vi "Calculate conductance slim.vi"(0 "File or Folder Path":path=path "P:/expt/Leiden MNK/SA02836H.20170110/47", 5 "single ended?":bool=TRUE, 7 "index":T1={"N1"=18, "N2"=19, "N3"=4, "N4"=5, "V1"=8, "V2"=10, "V3"=10, "V4"=13, "CURRENT"=12, "Vsg"=1}, 9 "offset":i32, 11 "length":i32=1000) -> (4 "A vs D":cluster{dbl[], dbl[]}[](graph))   [LabVIEW 2016]
panel:
  in  "e^2/h":bool=TRUE
  out "Path":path=path "P:/expt/Leiden MNK/SA02836H.20170110/47/47 - Sweep axis 1,2 - 1/SA02836H.20170110.000034.itx"
  in  "file contains 2D data?":bool
  in  "recolor traces?":bool
  in  "B x name":string="Vsg (V)"
  in  "A y name":string="Conductance (S)"
  in  "Generate Folder Index File?":bool
  in  "pattern":string="*.itx"
  in  "Use Folder Index File?":bool
  # "CURRENT/(V1-V2)"
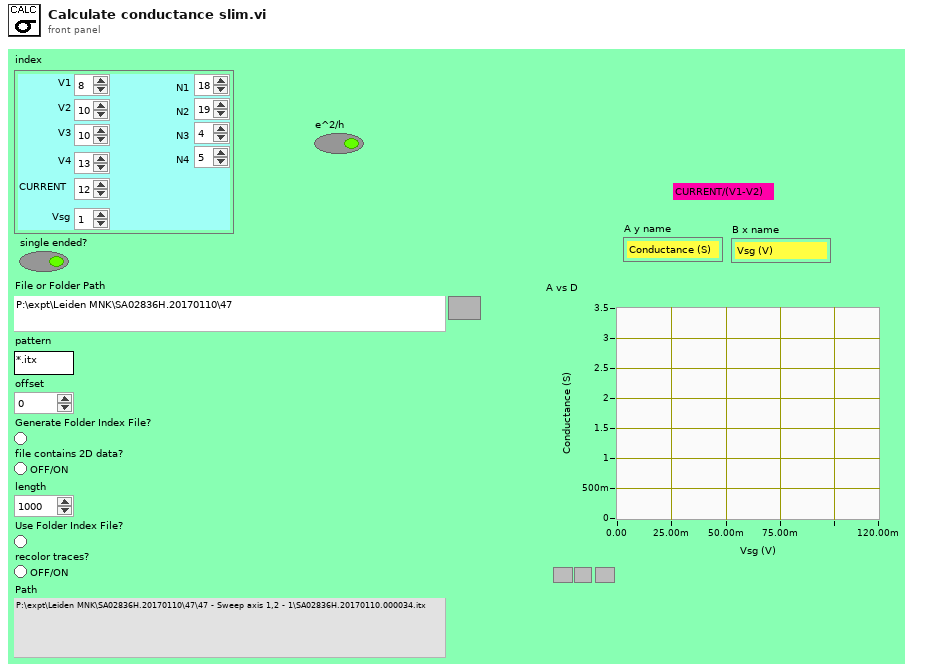
[diagram p1: front panel]
types:
  T1 = cluster{"N1":i32, "N2":i32, "N3":i32, "N4":i32, "V1":i32, "V2":i32, "V3":i32, "V4":i32, "CURRENT":i32, "Vsg":i32}
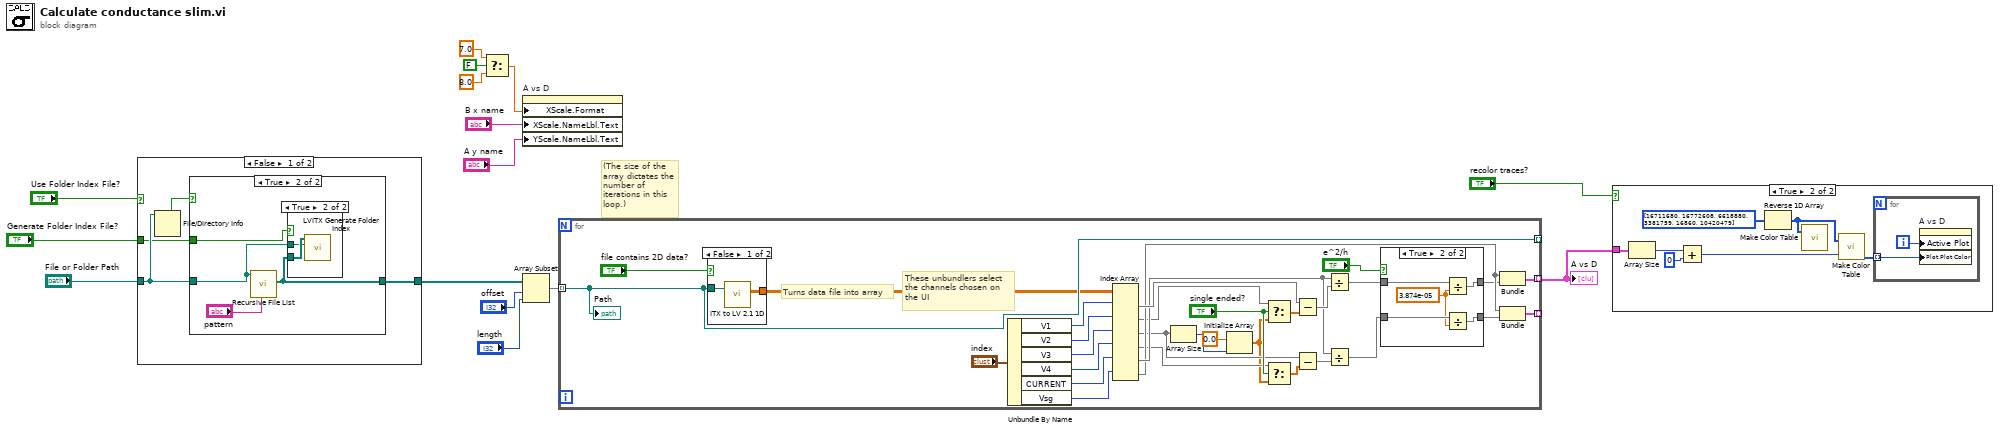
[diagram p0: block diagram]
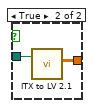
[diagram p4: hidden frame]
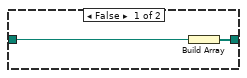
[diagram p5: hidden frame]
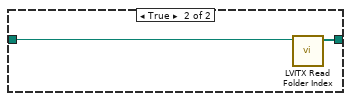
[diagram p7: hidden frame]
diagram:
  # "(The size of the array dictates the number of\niterations in this loop.)"
  n1 = case shown="False" "Use Folder Index File?" {
    tunnel: [w17 w28] -> w13
    tunnel: "File or Folder Path" -> [w19 w29]
    tunnel: "Generate Folder Index File?" -> [w16 _]
    frame False {
      n2 = File/Directory Info(path=w19) -> (directory=w18:bool)  [unwired: 1 in, 6 out]
      n3 = case shown="True" w18 {
        tunnel: [w21 w24] -> w17
        tunnel: w19 -> [w20 w23]
        tunnel: w16 -> [_ w22]
        frame False {
          n4 = Build Array(w20) -> (w21:path[])
        }
        frame True {
          n5 = call <vilib>:"Recursive File List.vi"("pattern"="pattern", "Folder Path"=w23) -> ("All Files in Dir"=w24:path[])  [unwired: 5 in, 4 out]
          n6 = case shown="True" w22 {
            tunnel: w24 -> [_ w27]
            tunnel: w23 -> [_ w26]
            frame False {
            }
            frame True {
              n7 = call <userlib>:"LVITX Generate Folder Index.vi"("File or Folder Path"=w26, "All Files in Dir"=w27) -> ()  [unwired: 10 in]
            }
          }
        }
      }
    }
    frame True {
      n8 = call <userlib>:"LVITX Read Folder Index.vi"("File or Folder Path"=w29) -> ("Array"=w28:path[])  [unwired: 10 in]
    }
  }
  n9 = Select(t=7.0, s=FALSE ("B is time?"), f=8.0) -> (s? t:f=w3:dbl)
  n10 = property on="A vs D" class="XYGraph (strict)"("XScale.Format"=w3, "XScale.NameLbl.Text"="B x name", "YScale.NameLbl.Text"="A y name") -> ()  [unwired: 2 in, 2 out]
  n11 = Array Subset(array=w13, index="offset", length="length") -> (w6:path[])
  n12 = for {
    tunnel: w6 -> [w60] mode=indexing
    tunnel: [w60] -> _ mode=indexing
    tunnel: [w31] -> w1 mode=indexing
    tunnel: [w47] -> _ mode=indexing
    # "These unbundlers select\nthe channels chosen on\nthe UI"
    # "Turns data file into array"
    n13 = case shown="False" "file contains 2D data?" {
      tunnel: [w68 w70] -> w52
      tunnel: w60 -> [w69 w71]
      frame False {
        n14 = call <userlib>:"ITX to LV 2.1 1D.vi"("file (use dialog)"=w69) -> ("1D arrays"=w68:dbl[][])  [unwired: 2 in, 2 out]
      }
      frame True {
        n15 = call <userlib>:"ITX to LV 2.1.vi"("file (use dialog)"=w71) -> ("1D arrays"=w70:dbl[][])  [unwired: 1 in, 3 out]
      }
    }
    n16 = Unbundle By Name("index") -> ("V1"=w57:i32, "V2"=w56:i32, "V3"=w55:i32, "V4"=w54:i32, "CURRENT"=w51:i32, "Vsg"=w46:i32)
    n17 = Index Array(array=w52, index (row) #1=w57, index (row) #2=w56, index (row) #3=w55, index (row) #4=w54, index (row) #5=w51, index (row) #6=w46) -> (element #1=w53:dbl[], element #2=w39:dbl[], element #3=w35:dbl[], element #4=w37:dbl[], element #5=w49:dbl[], element #6=w45:dbl[])  [unwired: 6 in]
    n18 = Array Size(array=w35) -> (size(s)=w33:i32)
    n19 = Initialize Array(0.0 ("element"), w33) -> (w32:dbl[])
    n20 = Select(t=w39, s="single ended?", f=w32) -> (s? t:f=w38:dbl[])
    n21 = Select(t=w37, s="single ended?", f=w32) -> (s? t:f=w36:dbl[])
    n22 = Subtract(x=w53, y=w38) -> (x-y=w50:dbl[])
    n23 = Subtract(x=w35, y=w36) -> (x-y=w48:dbl[])
    n24 = Divide(x=w49, y=w50) -> (x/y=w43:dbl[])
    n25 = Divide(x=w49, y=w48) -> (x/y=w44:dbl[])
    n26 = case shown="True" "e^2/h" {
      tunnel: w44 -> [w61 w65]
      tunnel: w43 -> [w62 w67]
      tunnel: [w62 w66] -> w41
      tunnel: [w61 w64] -> w42
      frame False {
      }
      frame True {
        w63 = 3.874e-05
        n27 = Divide(x=w67, y=w63) -> (x/y=w66:dbl[])
        n28 = Divide(x=w65, y=w63) -> (x/y=w64:dbl[])
      }
    }
    n29 = Bundle("1D arrays"=w45, w41) -> (w31:cluster{"1D arrays":dbl[], dbl[]})  [unwired: 1 in]
    n30 = Bundle("1D arrays"=w45, w42) -> (w47:cluster{"1D arrays":dbl[], dbl[]})  [unwired: 1 in]
    "Path" <- w60
  }
  "A vs D" <- w1
  n31 = case shown="True" "recolor traces?" {
    tunnel: w1 -> [_ w72]
    frame False {
    }
    frame True {
      n32 = Array Size(array=w72) -> (size(s)=w75:i32)
      n33 = Add(x=w75, y=0 ("x")) -> (x+y=w78:i32)
      n34 = Reverse 1D Array(array=u32[] [16711680, 16772608, 6618880, 3381759, 16860, 10420479] ("color scale")) -> (reversed array=w74:u32[])
      n35 = call <userlib>:"Make Color Table.vi"("Array"=w74) -> ()  [unwired: 1 in, 4 out]
      n36 = call <userlib>:"Make Color Table.vi"("Array"=w74, "Size/3"=w78) -> ("Color Tbl"=w76:u32[])  [unwired: 3 out]
      n37 = for {
        tunnel: w76 -> [w79] mode=indexing
        i -> [w80]
        n38 = property on="A vs D" class="XYGraph (strict)"("Active Plot"=w80, "Plot.Plot Color"=w79) -> ()  [unwired: 2 in, 2 out]
      }
    }
  }
